vi "Graph_Data.vi"() -> ()   [LabVIEW 2015]
uses:
  <vilib>/Utility/file.llb/Read Delimited Spreadsheet (DBL).vi
  <vilib>/Analysis/NI_AALPro.lvlib
  <vilib>/Analysis/NI_AALBase.lvlib
panel:
  in  "Constant Measurement":path
  out "Constant Rate":T1(graph)
  out "Decay Time (s)":dbl
  in  "Decay Measurement":path
  out "Decay Plot":cluster{dbl[], "Best Exponential Fit":dbl[]}[](graph)
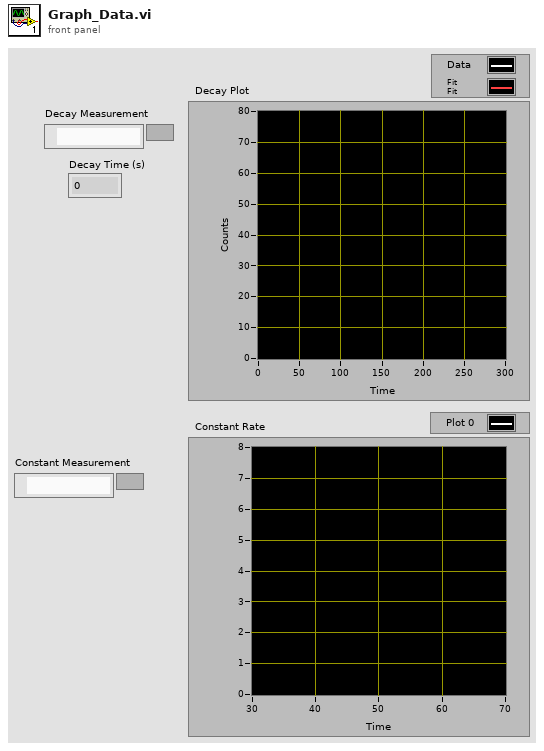
[diagram p1: front panel]
types:
  T1 = cluster{"X Values":dbl[], "Histogram: h(x)":i32[]}
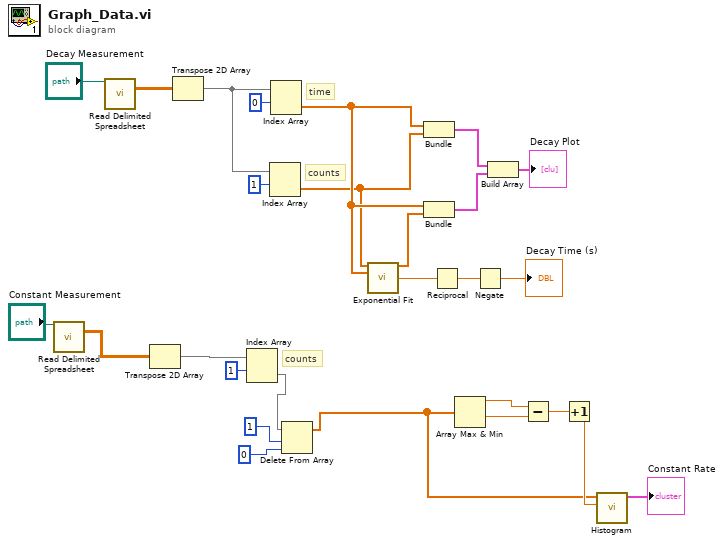
[diagram p0: block diagram]
diagram:
  # "counts"
  # "counts"
  # "time"
  n1 = call-poly <vilib>:"Read Delimited Spreadsheet.vi"("file path (dialog if empty)"="Constant Measurement") -> ("all rows"=w2:dbl[][])  [unwired: 9 in, 5 out]
  n2 = call-poly <vilib>:"Read Delimited Spreadsheet.vi"("file path (dialog if empty)"="Decay Measurement") -> ("all rows"=w26:dbl[][])  [unwired: 9 in, 5 out]
  n3 = Transpose 2D Array(2D array=w2) -> (transposed array=w6:dbl[][])
  n4 = Transpose 2D Array(2D array=w26) -> (transposed array=w23:dbl[][])
  n5 = Index Array(array=w6, index (row)=1) -> (element=w5:dbl[])  [unwired: 1 in]
  n6 = Index Array(array=w23, index (row)=1) -> (element=w14:dbl[])  [unwired: 1 in]
  n7 = Index Array(array=w23, index (row)=0) -> (element=w19:dbl[])  [unwired: 1 in]
  n8 = Delete From Array(array=w5, length=1, index=0) -> (array with subset deleted=w1:dbl[])  [unwired: 1 out]
  n9 = call <vilib>:"Exponential Fit.vi"("Y"=w14, "X"=w19) -> ("Best Exponential Fit"=w20:dbl[], "damping"=w17:dbl)  [unwired: 8 in, 4 out]
  n10 = Bundle(w19, w14) -> (w21:cluster{dbl[], dbl[]})  [unwired: 1 in]
  n11 = Bundle(w19, "Best Exponential Fit"=w20) -> (w22:cluster{dbl[], "Best Exponential Fit":dbl[]})  [unwired: 1 in]
  n12 = Reciprocal(x=w17) -> (1/x=w16:dbl)
  n13 = Array Max & Min(array=w1) -> (max value=w13:dbl, min value=w12:dbl)  [unwired: 2 out]
  n14 = Negate(x=w16) -> (-x=→"Decay Time (s)":dbl)
  n15 = Build Array(w21, w22) -> (→"Decay Plot":cluster{dbl[], "Best Exponential Fit":dbl[]}[])
  n16 = Subtract(x=w13, y=w12) -> (x-y=w11:dbl)
  n17 = Increment(x=w11) -> (x+1=w9:dbl)
  n18 = call <vilib>:"Histogram.vi"("intervals"=w9, "X"=w1) -> ("Histogram Graph"=→"Constant Rate":T1)  [unwired: 6 in, 3 out]
